vi "UNIST Get Active Job ID.vi"() -> ()   [LabVIEW 2020]
uses:
  <vilib>/Instr/_visa.llb/VISA Configure Serial Port (Instr).vi
panel:
  out "concatenated string":string
  out "error out":errorcluster
  out "read buffer":string
  in  "VISA resource name":refnum<visa-resource-name>
  in  "error in (no error)":errorcluster
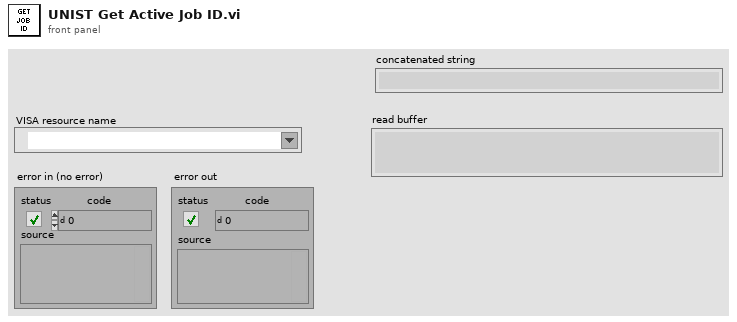
[diagram p1: front panel]
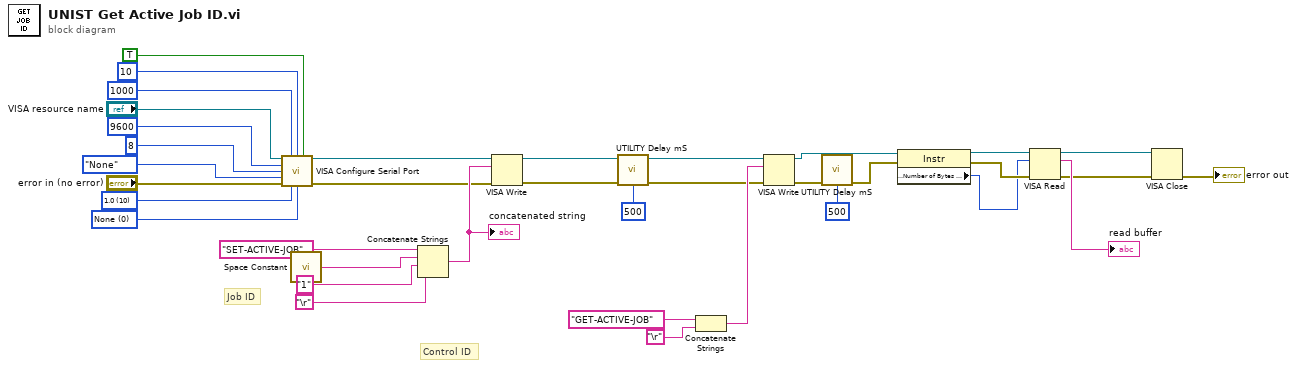
[diagram p0: block diagram]
diagram:
  w31 = u16 0 items=["None", "XON/XOFF", "RTS/CTS", "XON/XOFF & RTS/CTS", "DTR/DSR", "XON/XOFF & DTR/DSR"] ("flow control (0:none)")
  w30 = u16 10 items=["1.0"=10, "1.5"=15, "2.0"=20] ("stop bits (10: 1 bit)")
  # "Job ID"
  # "Control ID"
  n1 = call-poly "VISA Configure Serial Port"("VISA resource name"="VISA resource name", "timeout (10sec)"=u32 1000, "termination char\n(0xA = '\\n' = LF)"=u8 10 ("termination char\n(0xA = '\\n' = LF)"), "Enable Termination\nChar (T)"=TRUE ("Enable Termination\nChar (T)"), "baud rate (9600)"=u32 9600, "data bits (8)"=u16 8, "parity (0:none)"=enum16{"None", "Odd", "Even", "Mark", "Space"}."None", "error in (no error)"="error in (no error)", "stop bits (10: 1 bit)"=w30, "flow control (0:none)"=w31) -> ("VISA resource name out"=w4:refnum<visa-resource-name>, "error out"=w6:errorcluster)  [unwired: 4 in]
  n2 = call <vilib>:"Space Constant.vi"() -> ("String"=w7:string)
  n3 = Concatenate Strings("SET-ACTIVE-JOB" ("write buffer"), w7, "1" ("string"), "\r") -> (w11:string)
  "concatenated string" <- w11
  n4 = VISA Write(VISA resource name=w4, write buffer=w11, error in (no error)=w6) -> (VISA resource name out=w5:refnum<visa-resource-name>, error out=w2:errorcluster)  [unwired: 1 out]
  n5 = call "UTILITY Delay mS.vi"("Error In"=w2, "milliseconds to wait"=u32 500) -> ("Error Out"=w1:errorcluster)  [unwired: 13 in]
  n6 = Concatenate Strings("GET-ACTIVE-JOB" ("write buffer"), "\r") -> (w24:string)
  n7 = VISA Write(VISA resource name=w5, write buffer=w24, error in (no error)=w1) -> (VISA resource name out=w22:refnum<visa-resource-name>, error out=w13:errorcluster)  [unwired: 1 out]
  n8 = call "UTILITY Delay mS.vi"("Error In"=w13, "milliseconds to wait"=u32 500) -> ("Error Out"=w12:errorcluster)  [unwired: 13 in]
  n9 = property class="Instr"(reference=w22, error in=w12) -> (reference out=w21:refnum<visa-resource-name>, error out=w20:errorcluster, "Serial Settings:Number of Bytes at Serial Port"=w19:u32)
  n10 = VISA Read(VISA resource name=w21, byte count=w19, error in (no error)=w20) -> (VISA resource name out=w17:refnum<visa-resource-name>, read buffer=→"read buffer":string, error out=w16:errorcluster)  [unwired: 1 out]
  n11 = VISA Close(VISA resource name=w17, error in (no error)=w16) -> (error out=→"error out":errorcluster)
